vi "web scraper to API converter.vi"() -> (0 "error out":errorcluster)   [LabVIEW 2024]
uses:
  <vilib>/addons/_JKI.lib/Serialization/JSON/JKI JSON Serialization.lvlib
  CV_RESTful_Library/CV_RESTful_Lib.lvlib
  CV_RESTful_Library/typedefs/local_volume--cluster.ctl
  CV_Shared_Library/volume.type--enum.ctl
  CV_Shared_Library/CV_Shared_Library.lvlib
  <vilib>/addons/_JKI.lib/REST Client/classes/REST Client/REST Client.lvclass
panel:
  in  "Delay Time (s)":dbl
  out "progress":i32(slide) caption="403 of 2850" scale=0.0..2850.0
  out "current file":string
  in  "dest directory":path=path "D:/Comics/data/comicvine"
  in  "old scraper directory":path=path "D:/Comics/data/comicvine"
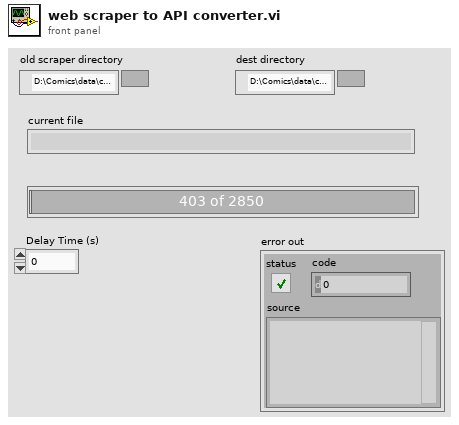
[diagram p1: front panel]
types:
  T1 = enum16{"open", "replace", "create", "open or create", "replace or create", "replace or create with confirmation"}
  T2 = typedef "CV_RESTful_Lib.lvlib/local_volume.ctl" = cluster{"id":i32, "name":string, "sortable_name":string, "aliases":string[], "description":string, "site_detail_url":string, "count_of_issues":i32, "start_year":i32, "publisher_id":i32, "issue_ids":i32[], "date_last_updated":timestamp, "volume":i32, "cv_id":string, "volume type":T3}
  T3 = typedef "CV_Shared_Library.lvlib/volume.type--enum.ctl" = enum16{"Ongoing", "Limited Series", "Annual", "One Shot", "Reprint/Document", "Star Comics", "Epic Comics"}
  T4 = typedef "CV_RESTful_Lib.lvlib/local_volume--cluster.ctl" = cluster{"id":i32, "name":string, "sortable_name":string, "aliases":string[], "description":string, "site_detail_url":string, "count_of_issues":i32, "start_year":i32, "publisher_id":i32, "issue_ids":i32[], "date_last_updated":timestamp, "volume":i32, "cv_id":string, "volume type":T3}
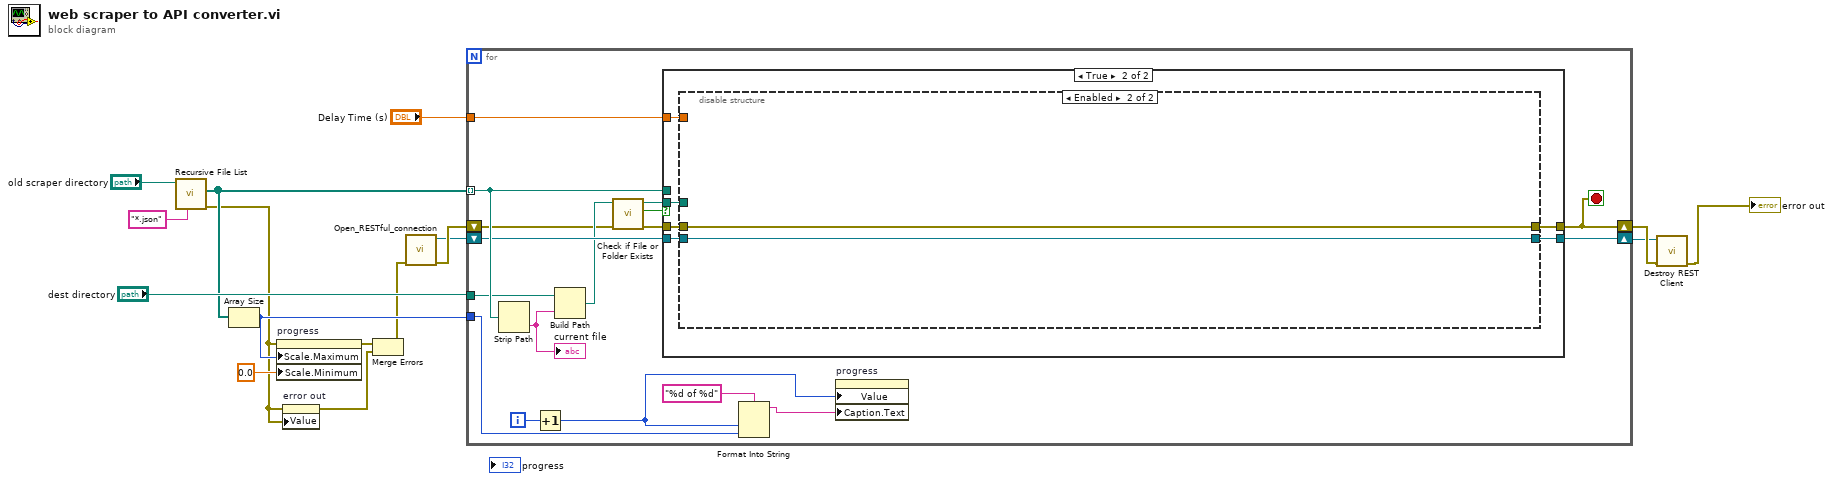
[diagram p0: block diagram]
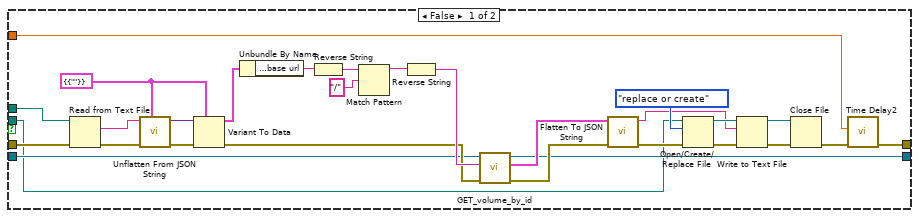
[diagram p2: hidden frame]
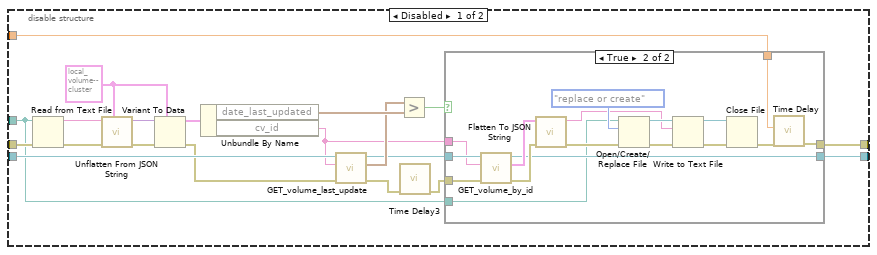
[diagram p3: hidden frame]
diagram:
  n1 = call <vilib>:"Recursive File List.vi"("pattern"="*.json", "Folder Path"="old scraper directory") -> ("error out"=w8:errorcluster, "All Files in Dir"=w10:path[])  [unwired: 5 in, 3 out]
  n2 = Array Size(array=w10) -> (size(s)=w9:i32)
  n3 = property on="progress" class="Slide (strict)"(error in=w8, "Scale.Maximum"=w9, "Scale.Minimum"=0.0 ("Scale.Range:Minimum")) -> (error out=w7:errorcluster)  [unwired: 1 in, 1 out]
  n4 = property on="error out" class="Clust (strict)"(error in=w8, "Value"=w8) -> (error out=w6:errorcluster)  [unwired: 1 in, 1 out]
  n5 = Merge Errors(w7, w6) -> (w5:errorcluster)
  n6 = call "Open_RESTful_connection.vi"("error in (no error)"=w5) -> ("error out"=w14:errorcluster, "REST Client out"=w12:refnum<class "REST Client.lvclass">)  [unwired: 9 in]
  n7 = for {
    tunnel: w10 -> [w33] mode=indexing
    shift-right: [w18] -> w3
    shift-left: w14 -> [w26]
    tunnel: "dest directory" -> [w32]
    shift-right: [w29] -> w1
    shift-left: w12 -> [w30]
    tunnel: w9 -> [w22]
    tunnel: "Delay Time (s)" -> [w17]
    i -> [w21]
    stop <- w18 stop-if-true
    n8 = Strip Path(path=w33) -> (name=w31:string)  [unwired: 1 out]
    "current file" <- w31
    n9 = Increment(x=w21) -> (x+1=w19:i32)
    n10 = Build Path(base path=w32, name or relative path=w31) -> (appended path=w28:path)
    n11 = call <vilib>:"Check if File or Folder Exists.vi"("error in (no error)"=w26, "path"=w28) -> ("error out"=w25:errorcluster, "file or folder exists?"=w27:bool, "dup path"=w24:path)  [unwired: 7 in]
    n12 = case shown="True" w27 {
      tunnel: w25 -> [w62 w68]
      tunnel: w33 -> [w45 _]
      tunnel: [w35 w65] -> w18
      tunnel: w30 -> [w39 w67]
      tunnel: [w38 w66] -> w29
      tunnel: w24 -> [w37 w64]
      tunnel: w17 -> [w34 w63]
      frame False {
        w57 = cluster{"seriesInfo":cluster{"base url":string}} {"seriesInfo"={"base url"=""}}
        n13 = Read from Text File(file (use dialog)=w45, error in=w62) -> (text=w60:string, error out=w61:errorcluster)  [unwired: 2 in, 2 out]
        n14 = call <vilib>:"Unflatten From JSON String.vi"("Type and Defaults"=w57, "error in"=w61, "JSON String"=w60) -> ("error out"=w59:errorcluster, "Variant"=w58:variant)  [unwired: 7 in]
        n15 = Variant To Data(error in=w59, type=w57, Variant=w58) -> (data=w56:cluster{"seriesInfo":cluster{"base url":string}}, error out=w50:errorcluster)
        n16 = Unbundle By Name(w56) -> ("seriesInfo.base url"=w55:string)
        n17 = Reverse String(1:w55) -> (0:w54:string)
        n18 = Match Pattern(string=w54, regular expression="/") -> (before substring=w52:string)  [unwired: 1 in, 3 out]
        n19 = Reverse String(1:w52) -> (0:w51:string)
        n20 = call "GET_volume_by_id.vi"("error in (no error)"=w50, "volume id"=w51, "REST Client in"=w39) -> ("error out"=w48:errorcluster, "local volume"=w49:T2, "REST Client out"=w38:refnum<class "REST Client.lvclass">)  [unwired: 6 in]
        n21 = call <vilib>:"Flatten To JSON String.vi"("error in"=w48, "Variant"=w49) -> ("error out"=w46:errorcluster, "JSON String"=w42:string)  [unwired: 8 in]
        n22 = Open/Create/Replace File(file path (use dialog)=w37, error in=w46, operation (0:open)=T1."replace or create") -> (refnum out=w43:refnum<file>, error out=w44:errorcluster)  [unwired: 3 in, 1 out]
        n23 = Write to Text File(file (use dialog)=w43, text=w42, error in=w44) -> (refnum out=w40:refnum<file>, error out=w41:errorcluster)  [unwired: 1 in, 1 out]
        n24 = Close File(refnum=w40, error in=w41) -> (error out=w36:errorcluster)  [unwired: 1 out]
        n25 = call "Time Delay2"("error in (no error)"=w36, "Delay Time (s)"=w34) -> ("error out"=w35:errorcluster)  [unwired: 9 in]
      }
      frame True {
        n26 = disable-structure shown="Enabled" {
          disable-tunnel: w68 -> [w88 w108]
          disable-tunnel: w67 -> [w81 w109]
          disable-tunnel: [w74 w109] -> w66
          disable-tunnel: [w73 w108] -> w65
          disable-tunnel: w64 -> [w72 _]
          disable-tunnel: w63 -> [w71 _]
          frame Disabled {
            w82 = T4 {"id"=0, "name"="", "sortable_name"="", "aliases"=[], "description"="", "site_detail_url"="", "count_of_issues"=0, "start_year"=0, "publisher_id"=0, "issue_ids"=[], "date_last_updated"=timestamp(0 s since 1904-01-01), "volume"=0, "cv_id"="", "volume type"=enum."One Shot"} ("local volume")
            n27 = Read from Text File(file (use dialog)=w72, error in=w88) -> (text=w87:string, error out=w84:errorcluster)  [unwired: 2 in, 2 out]
            n28 = call <vilib>:"Unflatten From JSON String.vi"("Type and Defaults"=w82, "error in"=w84, "JSON String"=w87) -> ("error out"=w86:errorcluster, "Variant"=w85:variant)  [unwired: 7 in]
            n29 = Variant To Data(error in=w86, type=w82, Variant=w85) -> (data=w83:T4, error out=w80:errorcluster)
            n30 = Unbundle By Name(w83) -> ("date_last_updated"=w79:timestamp, "cv_id"=w75:string)
            n31 = call "GET_volume_last_update.vi"("error in (no error)"=w80, "volume id"=w75, "REST Client in"=w81) -> ("error out"=w70:errorcluster, "results.date_last_updated"=w78:timestamp, "REST Client out"=w76:refnum<class "REST Client.lvclass">)  [unwired: 6 in]
            n32 = Greater?(x=w78, y=w79) -> (0:w77:bool)
            n33 = call "Time Delay3"("error in (no error)"=w70) -> ("error out"=w69:errorcluster)  [unwired: 10 in]
            n34 = case shown="True" w77 {
              tunnel: w76 -> [w89 w107]
              tunnel: w69 -> [w90 w106]
              tunnel: w75 -> [_ w105]
              tunnel: [w89 w96] -> w74
              tunnel: [w90 w92] -> w73
              tunnel: w72 -> [_ w94]
              tunnel: w71 -> [_ w91]
              frame False {
              }
              frame True {
                n35 = call "GET_volume_by_id.vi"("error in (no error)"=w106, "volume id"=w105, "REST Client in"=w107) -> ("error out"=w98:errorcluster, "local volume"=w97:T2, "REST Client out"=w96:refnum<class "REST Client.lvclass">)  [unwired: 6 in]
                n36 = call <vilib>:"Flatten To JSON String.vi"("error in"=w98, "Variant"=w97) -> ("error out"=w95:errorcluster, "JSON String"=w99:string)  [unwired: 8 in]
                n37 = Open/Create/Replace File(file path (use dialog)=w94, error in=w95, operation (0:open)=T1."replace or create") -> (refnum out=w103:refnum<file>, error out=w104:errorcluster)  [unwired: 3 in, 1 out]
                n38 = Write to Text File(file (use dialog)=w103, text=w99, error in=w104) -> (refnum out=w101:refnum<file>, error out=w102:errorcluster)  [unwired: 1 in, 1 out]
                n39 = Close File(refnum=w101, error in=w102) -> (error out=w93:errorcluster)  [unwired: 1 out]
                n40 = call "Time Delay"("error in (no error)"=w93, "Delay Time (s)"=w91) -> ("error out"=w92:errorcluster)  [unwired: 9 in]
              }
            }
          }
          frame Enabled {
          }
        }
      }
    }
    n41 = Format Into String(format string="%d of %d", w19, w22) -> (resulting string=w20:string)  [unwired: 2 in, 1 out]
    n42 = property on="progress" class="Slide (strict)"("Value"=w19, "Caption.Text"=w20) -> ()  [unwired: 2 in, 2 out]
  }
  n43 = call-dynamic "Destroy REST Client.vi"("error in (no error)"=w3, "REST Client in"=w1) -> ("error out"=→"error out":errorcluster)  [unwired: 9 in]
